vi "Close Session.vi"(0 "eye scan in":refnum<class "niHighSpeedSerial N Point Eye Scan v1 Host.lvclass">, 11 "error in":errorcluster) -> (15 "error out":errorcluster)   [LabVIEW 2014, in "niHighSpeedSerial N Point Eye Scan v1 Host.lvclass"]
doc: "Closes the specified session and frees reserved resources. If the session is running, it is first aborted.\n\n<B>Input Parameters</B>\n\n<B>eye scan in</B> Takes in a reference to your session from the previous VI.\n\n<B>error in</B> describes error conditions that occur before this node runs. This input provides standard 'error in' functionality.\n\n<B>Output Parameters</B>\n\n<B>error out</B> contains error information. This output provides standard 'error out' functionality."
uses:
  <instrlib>/niHighSpeedSerial/Eye Scan/v1/Host/Impl/N Point Eye Scan/niHighSpeedSerial N Point Eye Scan v1 Host.lvclass
  <instrlib>/niHighSpeedSerial/Eye Scan/v1/Host/Eye Scan/niHighSpeedSerial Eye Scan v1 Host.lvclass
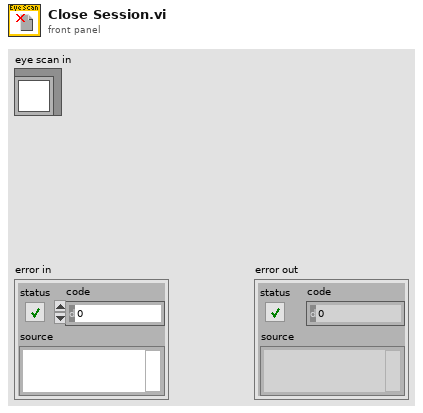
[diagram p1: front panel]
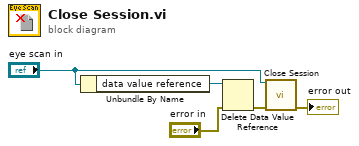
[diagram p0: block diagram]
diagram:
  n1 = Unbundle By Name("eye scan in") -> ("data value reference"=w3:refnum<data-value>)
  n2 = Delete Data Value Reference(data value reference=w3, error in="error in") -> (error out=w1:errorcluster)  [unwired: 1 out]
  n3 = call-parent "Close Session.vi"("eye scan in"="eye scan in", "error in"=w1) -> ("error out"=→"error out":errorcluster)  [unwired: 13 in]
